vi "UI.vi"(7 "Calculate":bool, 8 "Error In":errorcluster, 9 "B":dbl, 10 "A":dbl, 11 "Data Value Reference In":refnum<data-value>) -> (0 "Error Out":errorcluster, 2 "C":dbl, 3 "Data Value Reference Out":refnum<data-value>)   [LabVIEW 2021, in "Calculator.lvlib" / "Add.lvclass"]
doc: "This VI has two controls and a boolean in which the user enters input. When the calculate boolean is pressed the output is displayed in the indicator. This UI.vi is openend in the subpanel of main VI."
uses:
  Add.lvclass
  Calculator.lvlib
  Controls/User Event Operations.ctl
  NumericOperation/NumericOperation.lvclass
panel:
  # "Addition"
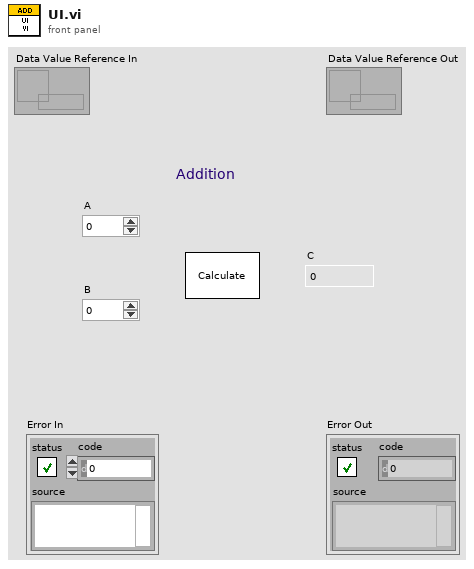
[diagram p1: front panel]
types:
  T1 = typedef "Calculator.lvlib/User Event Operations.ctl" = enum16{"Obtain", "Generate", "Release"}
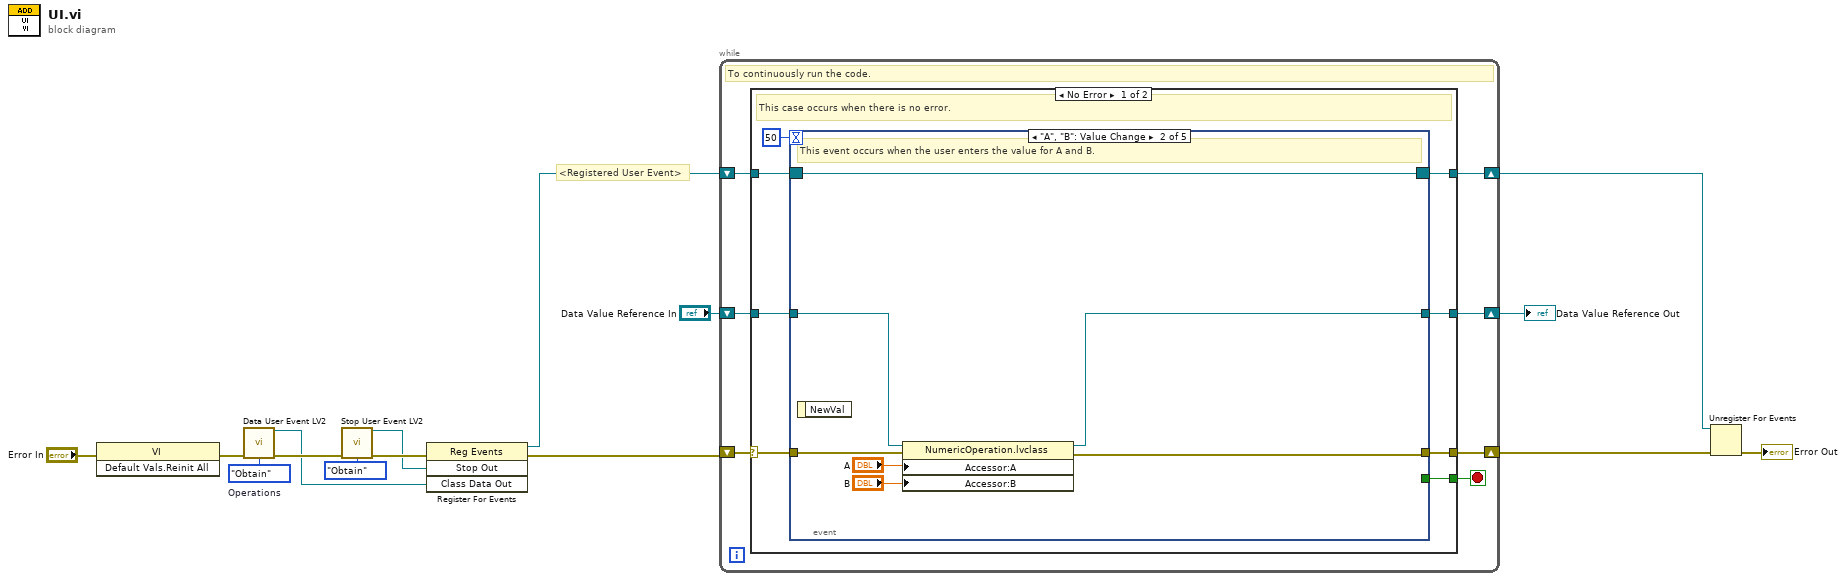
[diagram p0: block diagram]
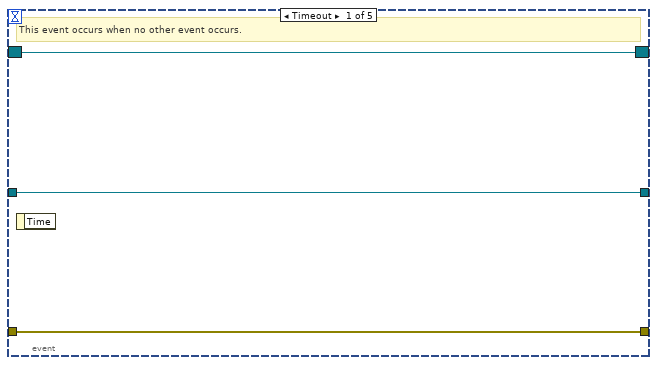
[diagram p2: hidden frame]
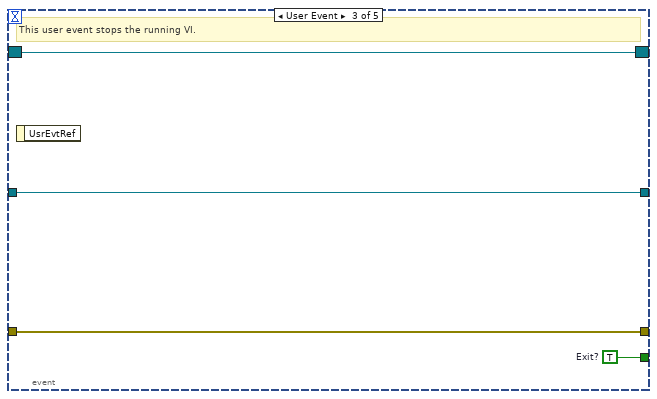
[diagram p3: hidden frame]
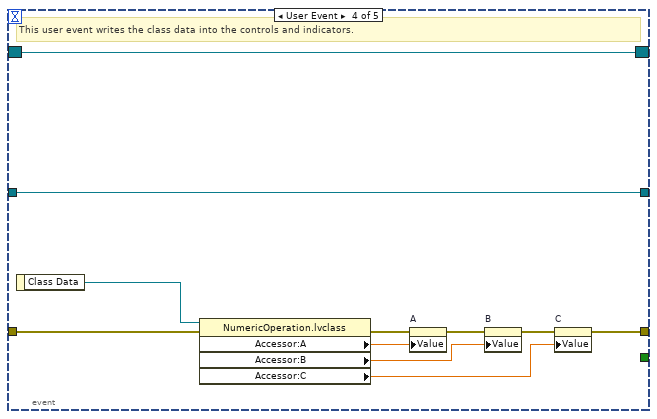
[diagram p4: hidden frame]
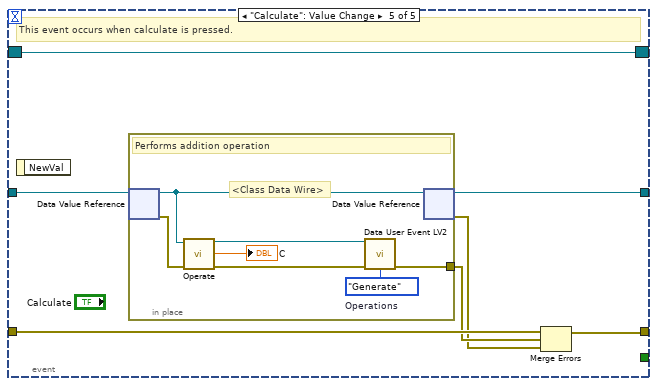
[diagram p5: hidden frame]
diagram:
  w3 = User_Event_Operations."Obtain"  # Operations
  # "<Registered User Event>"
  n1 = invoke class="VI" method="Default Vals.Reinit All"(error in="Error In") -> (error out=w8:errorcluster)  [unwired: 2 in, 2 out]
  n2 = call "Data User Event LV2.vi"("Error In"=w8, "Operations"=w3) -> ("Class Data Out"=w5:refnum<user-event>, "Error Out"=w9:errorcluster)  [unwired: 12 in]
  n3 = call "Stop User Event LV2.vi"("Error In"=w9, "Operations"=User_Event_Operations."Obtain") -> ("Stop Out"=w6:refnum<user-event>, "Error Out"=w7:errorcluster)  [unwired: 12 in]
  n4 = register-events(error in=w7, w6, w5) -> (reference out=w14:refnum<event-registration>, error out=w15:errorcluster)  [unwired: 1 in]
  n5 = while {
    shift-right: [w21] -> w13
    shift-left: w15 -> [w22]
    shift-right: [w19] -> w1
    shift-left: "Data Value Reference In" -> [w20]
    shift-right: [w16] -> w11
    shift-left: w14 -> [w18]
    stop <- w17 stop-if-true
    # "To continuously run the code."
    n6 = case shown="No Error" w22 {
      selector: w22 -> [w28 w72]
      tunnel: [w27 w72] -> w21
      tunnel: [w29 w71] -> w19
      tunnel: w20 -> [w30 w71]
      tunnel: w18 -> [w26 w70]
      tunnel: [w25 _] -> w17
      tunnel: [w23 w70] -> w16
      frame No Error {
        # "This case occurs when there is no error."
        n7 = event shown="[1] \"A\", \"B\": Value Change" {
          selector: w26 -> [w31 w34 w41 w45 w62]
          dyn-events: [w31 w34 w41 w45 w62] -> w23
          timeout: 50 -> [_ _ _ _ _]
          tunnel: [w33 w35 w44 w52 w60] -> w29
          tunnel: w30 -> [w33 w38 w44 w52 w61]
          tunnel: [w32 w39 w42 w49 w56] -> w27
          tunnel: w28 -> [w32 w40 w42 w55 w59]
          tunnel: [_ _ w43 _ _] -> w25
          event Timeout {
            # "This event occurs when no other event occurs."
            n8 = event-data() -> ()  [unwired: 1 in, 1 out]
          }
          event "A", "B": Value Change {
            # "This event occurs when the user enters the value for A and B."
            n9 = event-data() -> ()  [unwired: 1 in, 1 out]
            n10 = property class="NumericOperation.lvclass"(reference=w38, error in=w40, "Accessor:A"="A", "Accessor:B"="B") -> (reference out=w35:refnum<data-value>, error out=w39:errorcluster)
          }
          event User Event {
            w43 = TRUE  # Exit?
            # "This user event stops the running VI."
            n11 = event-data() -> ()  [unwired: 1 in, 1 out]
          }
          event User Event {
            # "This user event writes the class data into the controls and indicators."
            n12 = event-data() -> ("Class Data"=w54:refnum<class "NumericOperation.lvclass">)  [unwired: 1 in]
            n13 = property class="NumericOperation.lvclass"(reference=w54, error in=w55) -> (error out=w53:errorcluster, "Accessor:A"=w48:dbl, "Accessor:B"=w47:dbl, "Accessor:C"=w46:dbl)  [unwired: 1 out]
            n14 = property on="A" class="DigNum (strict)"(error in=w53, "Value"=w48) -> (error out=w51:errorcluster)  [unwired: 1 in, 1 out]
            n15 = property on="B" class="DigNum (strict)"(error in=w51, "Value"=w47) -> (error out=w50:errorcluster)  [unwired: 1 in, 1 out]
            n16 = property on="C" class="DigNum (strict)"(error in=w50, "Value"=w46) -> (error out=w49:errorcluster)  [unwired: 1 in, 1 out]
          }
          event "Calculate": Value Change {
            # "This event occurs when calculate is pressed."
            n17 = event-data() -> ()  [unwired: 1 in, 1 out]
            n18 = in-place {
              in-place-border: [w67] -> w58
              w66 = User_Event_Operations."Generate"  # Operations
              # "<Class Data Wire>"
              # "Performs addition operation"
              n19 = in-place-dvr #1(w61) -> (w64:refnum<class "NumericOperation.lvclass">, w63:errorcluster)
              n20 = call-dynamic "Operate.vi"("Error In"=w63, "NumericOperation in"=w64) -> ("Error Out"=w68:errorcluster, "C"=→"C":dbl, "NumericOperation out"=w65:refnum<class "NumericOperation.lvclass">)  [unwired: 7 in]
              n21 = call "Data User Event LV2.vi"("Class Data"=w65, "Error In"=w68, "Operations"=w66) -> ("Error Out"=w67:errorcluster)  [unwired: 11 in, 1 out]
              n22 = in-place-dvr #1(w64) -> (w60:refnum<data-value>, w57:errorcluster)
            }
            n23 = Merge Errors(w59, w58, w57) -> (w56:errorcluster)
          }
        }
      }
      frame Error {
        # "This case occurs when there is any error."
      }
    }
  }
  "Data Value Reference Out" <- w1
  n24 = Unregister For Events(event registration refnum=w11, error in=w13) -> (error out=→"Error Out":errorcluster)
